vi "TWO AXIS.vi"() -> ()   [LabVIEW 2014]
uses:
  Control 1.ctl
  <vilib>/Instr/_visa.llb/VISA Flush IO Buffer Mask.ctl
  <vilib>/Instr/_visa.llb/VISA Configure Serial Port (Instr).vi
panel:
  in  "?":bool
  in  "X Positions (0<X<95)":dbl[](array[numeric])
  in  "Y Positions (0<Y<88)":dbl[](array[numeric])
  # "End Command:\n10000"
  # "There can be no values after 10000, causes the motor to rotate infinitely. To delete a cell, \nright click on the cell, then select, Data Operations -> Delete Element. \n10000 MUST BE THE LAST COMMAND."
  # "All Values are in cm."
  # "System operates by moving to a given Y-Value,\nthen iterates through all X values. After all Y-Values\nare complete the program waits for user confirmation\nthen returns to (0,0)."
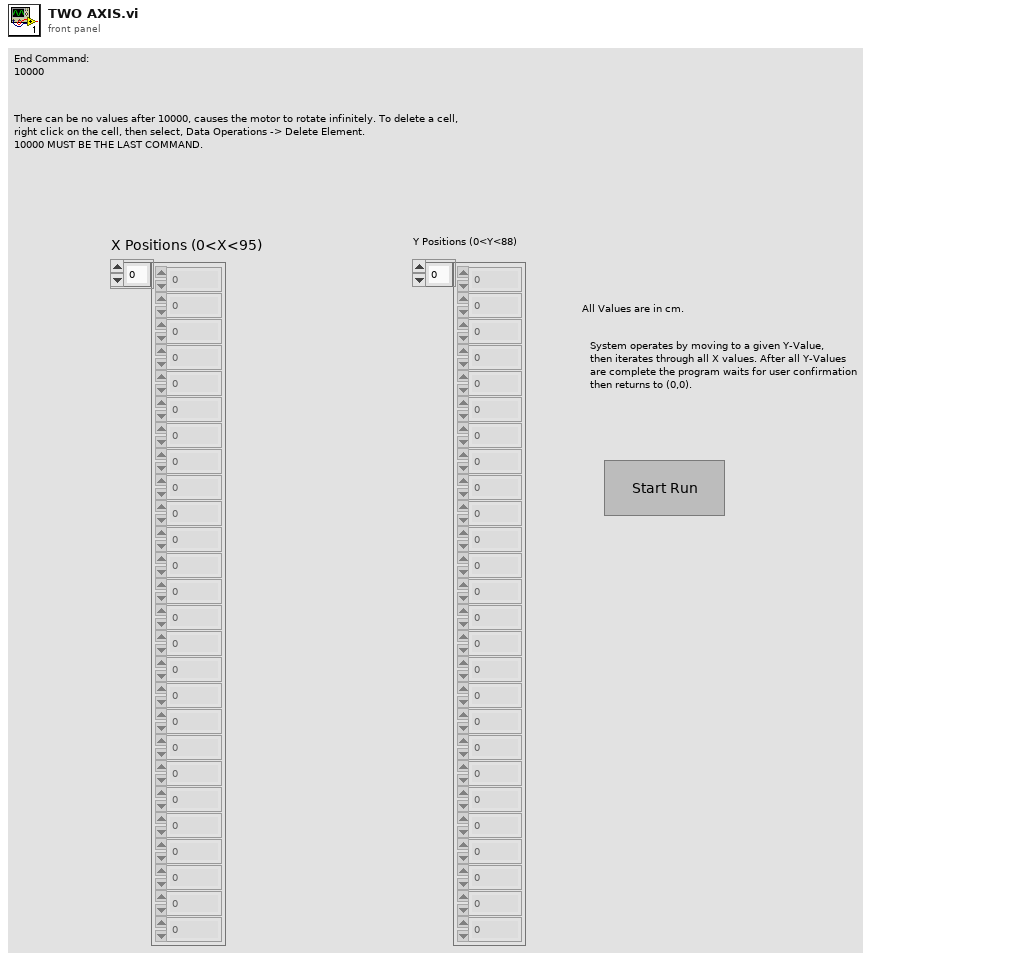
[diagram p1: front panel]
types:
  T1 = typedef "Control 1.ctl" = enum16{"Start", "Init", "Await Arduino Response", "Calculate Move", "Execute Move", "Home"}
  T2 = typedef "VISA Flush IO Buffer Mask.ctl" = u16
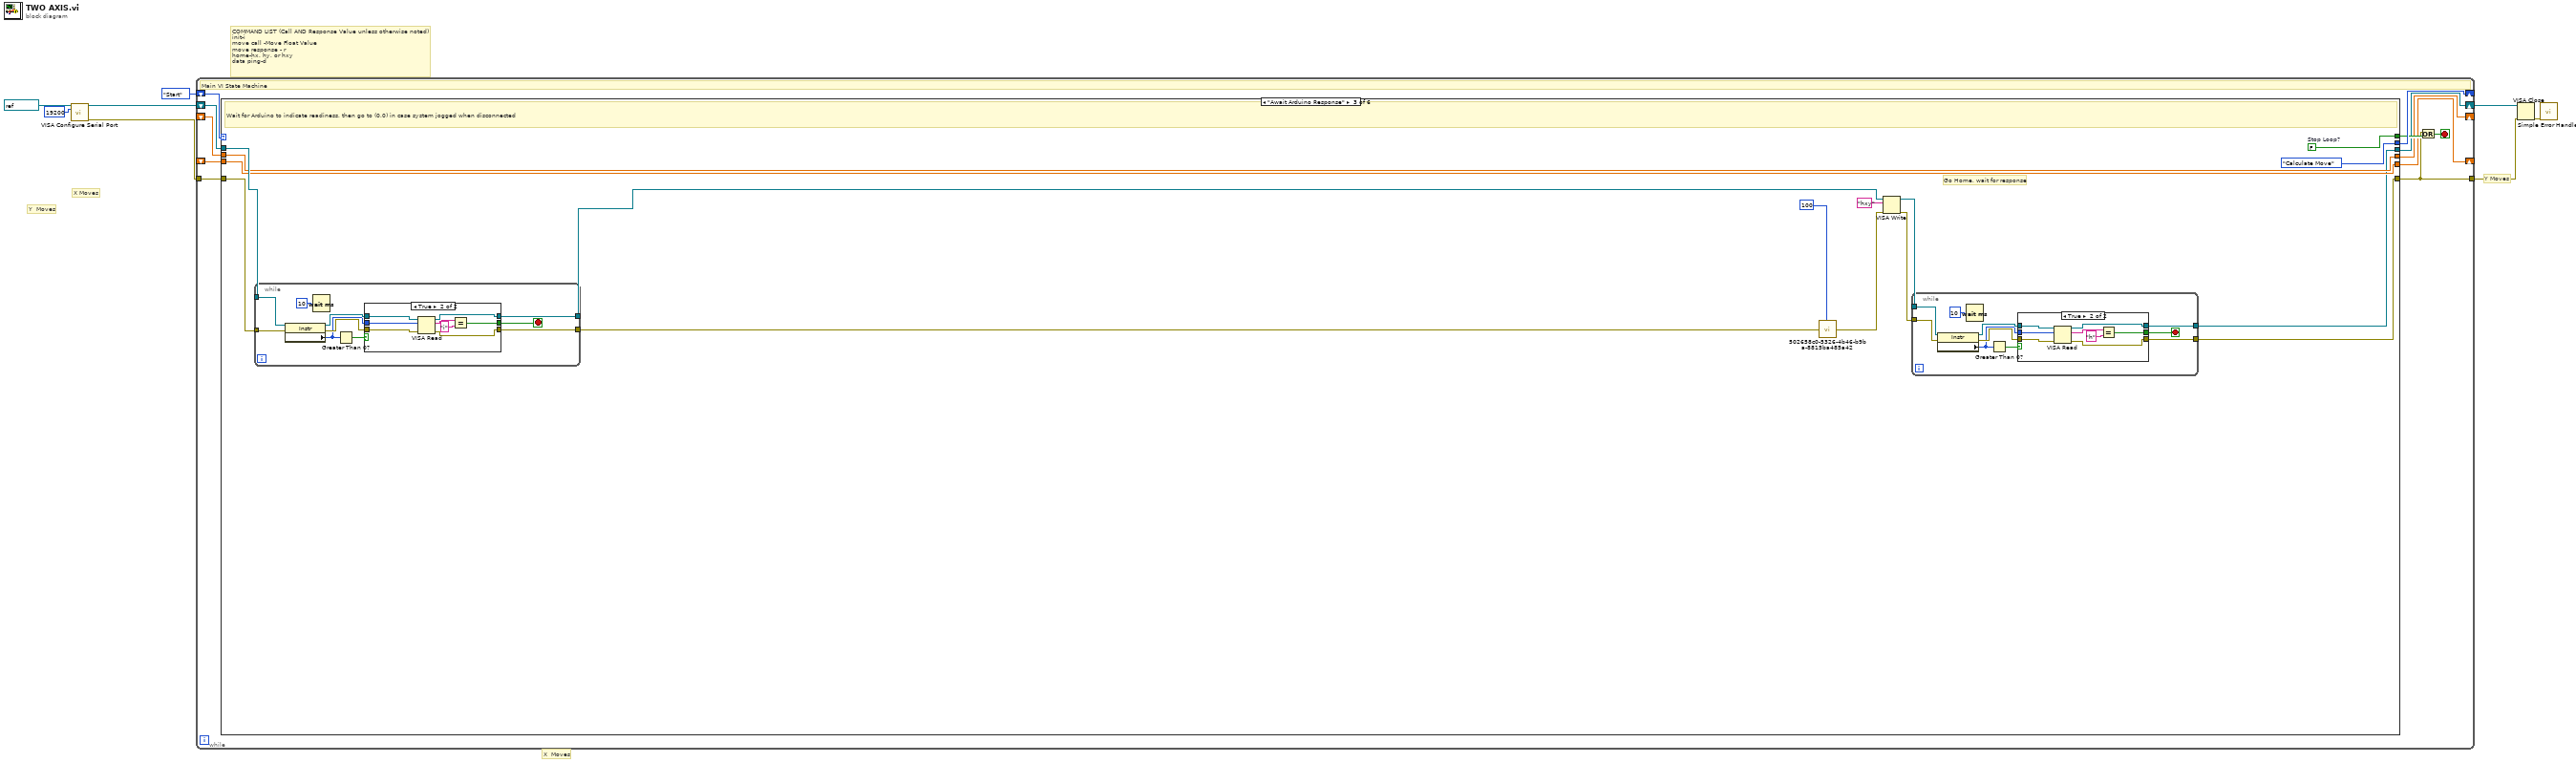
[diagram p0: block diagram]
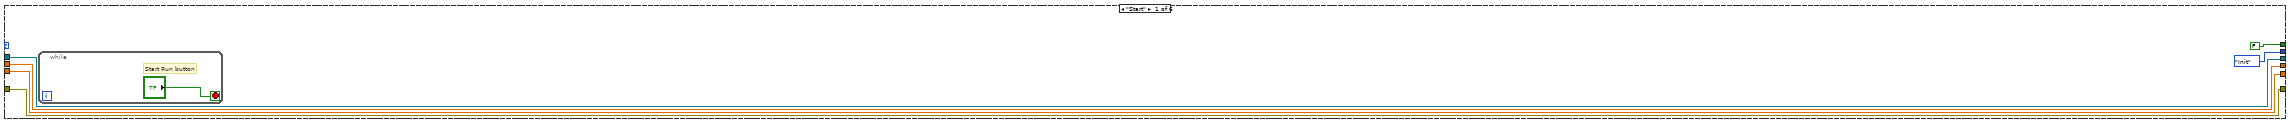
[diagram p2: hidden frame]
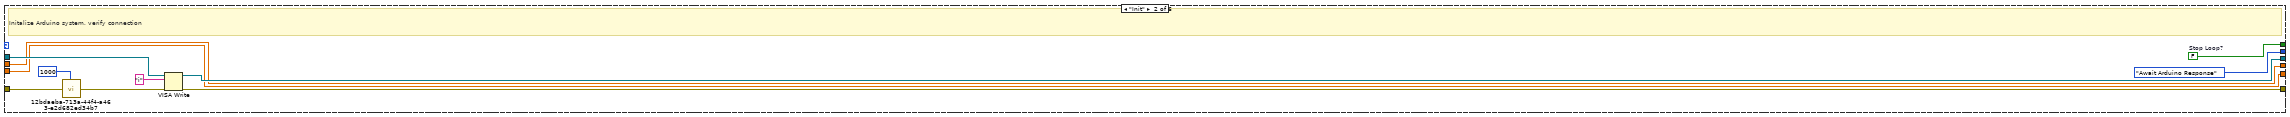
[diagram p3: hidden frame]
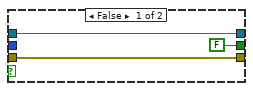
[diagram p4: hidden frame]
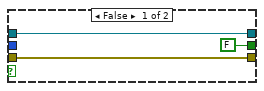
[diagram p5: hidden frame]
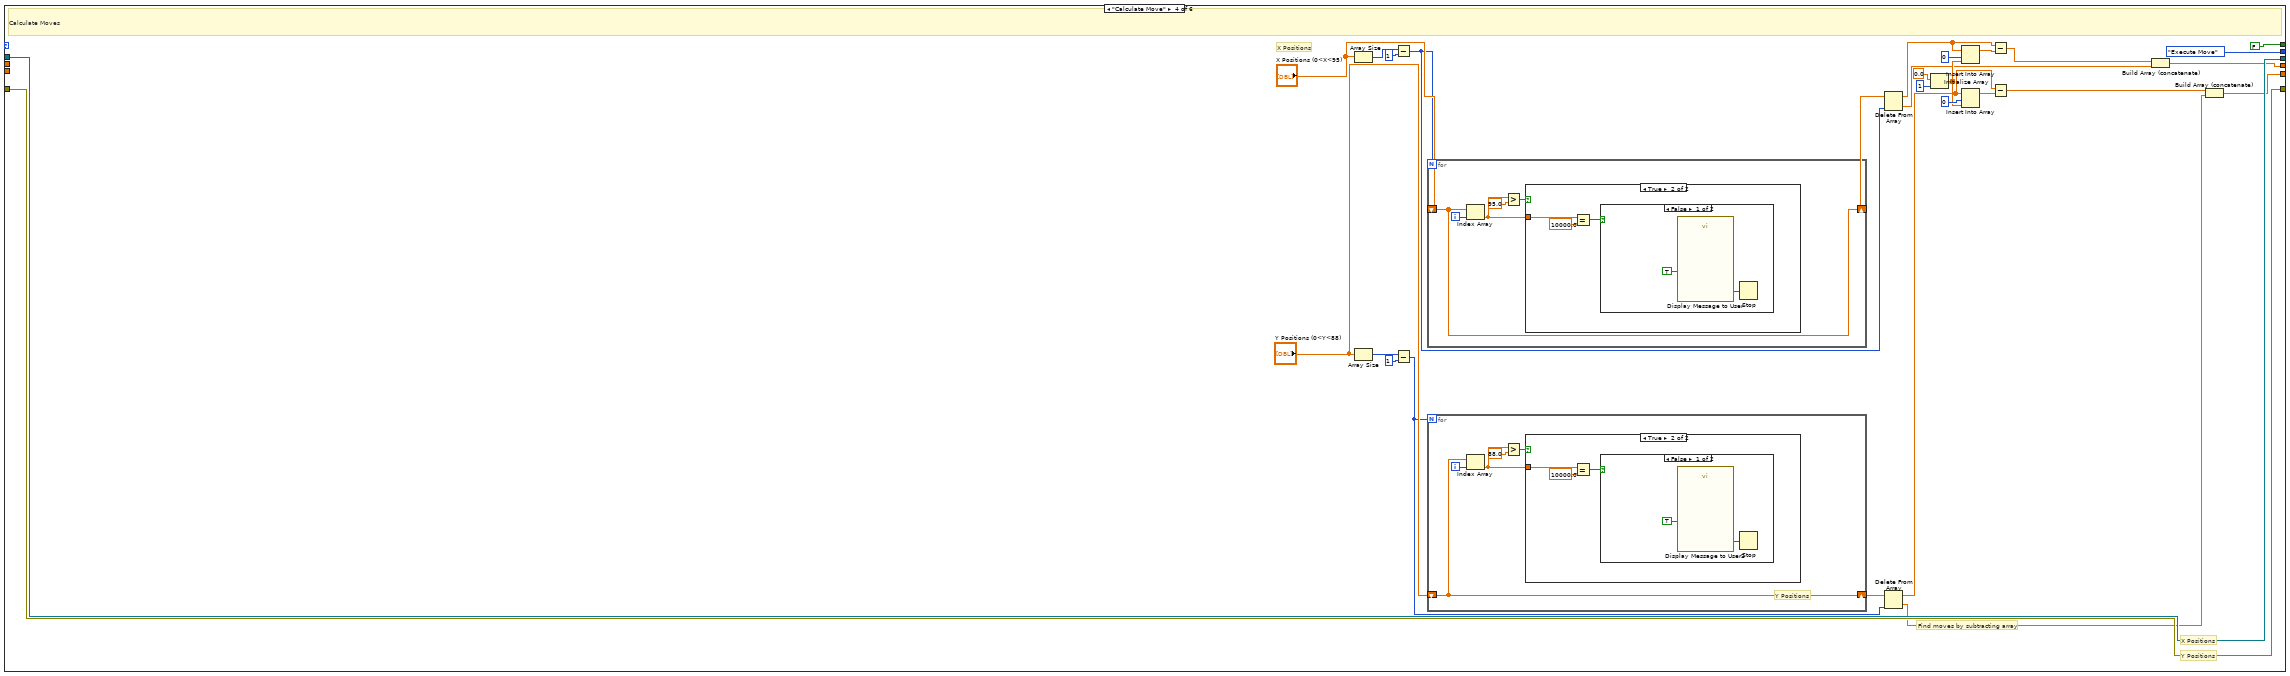
[diagram p6: hidden frame]
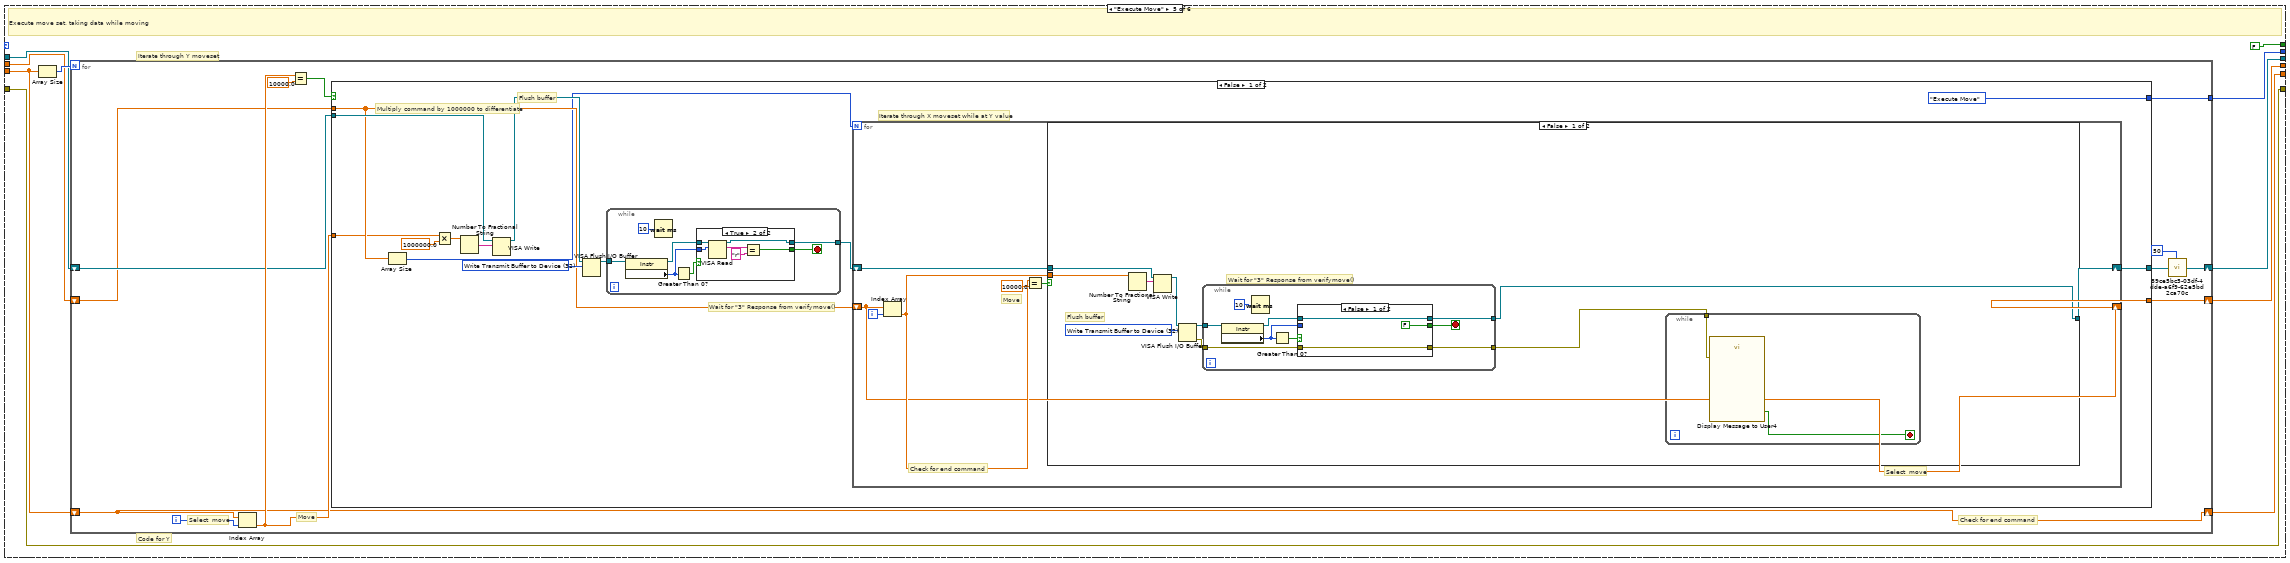
[diagram p11: hidden frame]
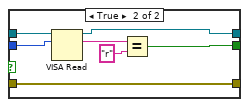
[diagram p12: hidden frame]
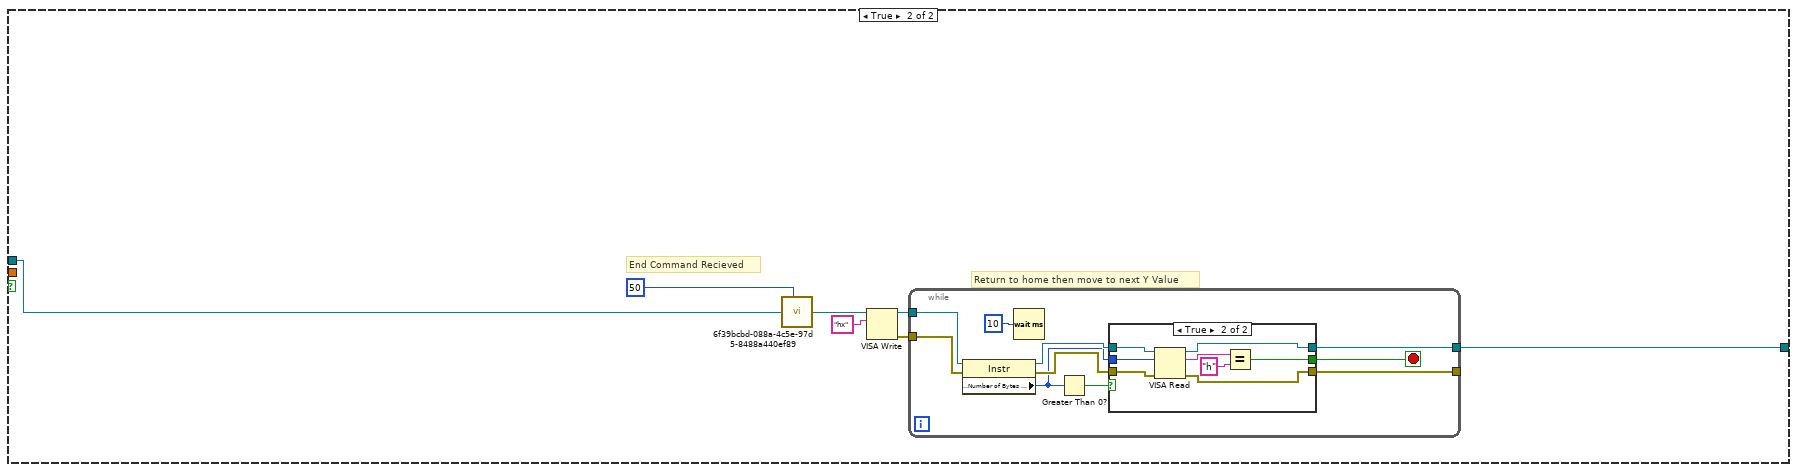
[diagram p13: hidden frame]
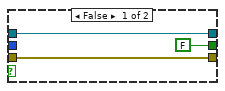
[diagram p14: hidden frame]
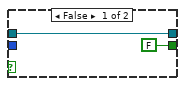
[diagram p15: hidden frame]
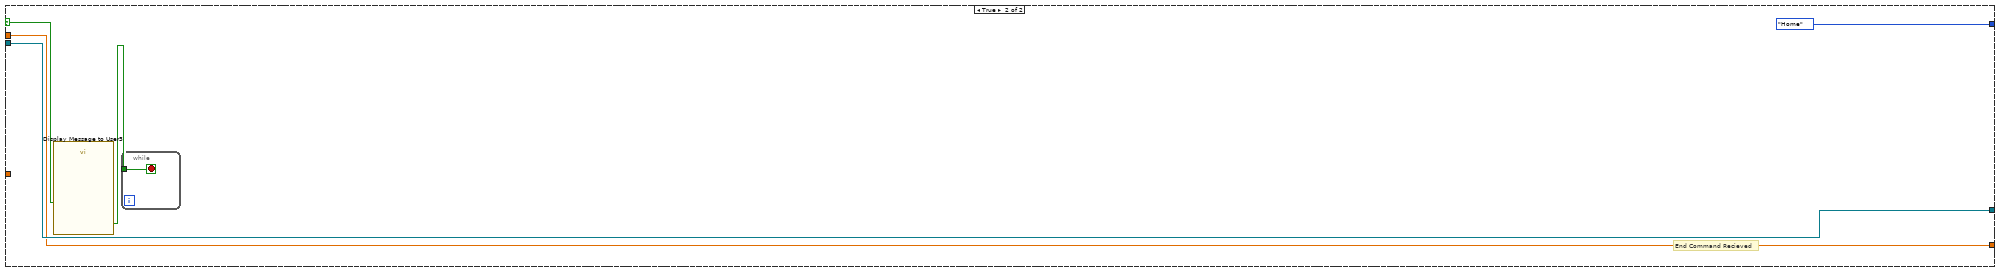
[diagram p16: hidden frame]
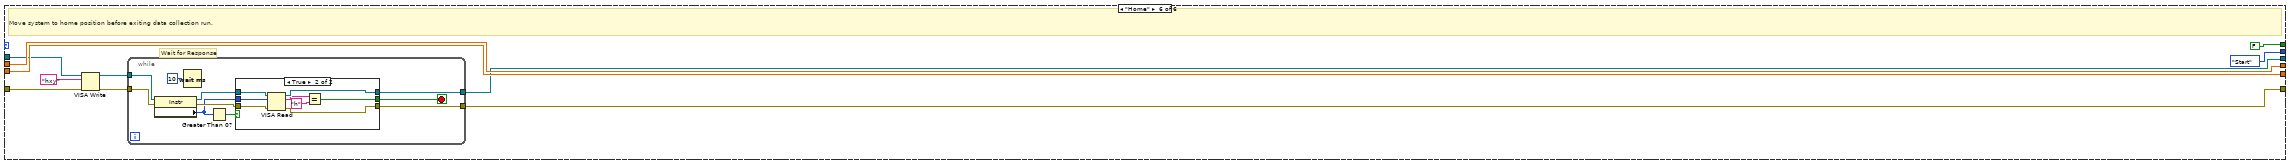
[diagram p17: hidden frame]
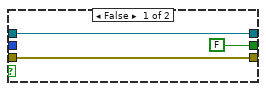
[diagram p18: hidden frame]
diagram:
  # "X  Moves"
  # "COMMAND LIST (Call AND Response Value unless otherwise noted)\ninit-i\nmove call -Move Float Value\nmove response - r\nhome-hx, hy, or hxy\ndata ping-d"
  # "Y Moves"
  # "X Moves"
  # "Y  Moves"
  n1 = call-poly "VISA Configure Serial Port"("VISA resource name"=refnum<visa-resource-name> "COM9", "baud rate (9600)"=u32 19200) -> ("VISA resource name out"=w6:refnum<visa-resource-name>, "error out"=w2:errorcluster)  [unwired: 12 in]
  n2 = while {
    shift-right: [w19] -> _
    shift-left: Control_1."Start" -> [w20]
    shift-right: [w16] -> w5
    shift-left: w6 -> [w17]
    shift-right: [w15] -> _
    shift-left: _ -> [w13]
    shift-right: [w14] -> _
    shift-left: _ -> [w12]
    tunnel: w2 -> [w11]
    tunnel: [w10] -> w1
    stop <- w9 stop-if-true
    # "Main VI State Machine"
    n3 = case shown="\"Await Arduino Response\"" w20 {
      tunnel: [Control_1."Init" Control_1."Await Arduino Response" Control_1."Calculate Move" Control_1."Execute Move" w148 Control_1."Start"] -> w19
      tunnel: [FALSE ("Stop Loop?") w38 w53 FALSE FALSE FALSE ("Stop Loop?")] -> w18
      tunnel: w17 -> [w23 w32 w52 w122 w145 w273]
      tunnel: w11 -> [w24 w34 w51 w121 w149 w272]
      tunnel: [w23 w35 w40 w122 w150 w268] -> w16
      tunnel: [w24 w36 w39 w121 w149 w267] -> w10
      tunnel: [w26 w29 w49 w104 w146 w275] -> w15
      tunnel: [w25 w28 w48 w103 w151 w274] -> w14
      tunnel: w13 -> [w26 w29 w49 _ w147 w275]
      tunnel: w12 -> [w25 w28 w48 _ w152 w274]
      frame "Start" {
        n4 = while {
          stop <- "?" stop-if-true
          # "Start Run button"
        }
      }
      frame "Init" {
        w38 = FALSE  # Stop Loop?
        # "Initalize Arduino system, verify connection"
        n5 = call "12bdaeba-713a-44f4-a463-e2d682ed34b7.vi"("value in"=w34, "milliseconds to wait"=u32 1000) -> ("value out"=w33:errorcluster)  [unwired: 1 out]
        n6 = VISA Write(VISA resource name=w32, write buffer="i", error in (no error)=w33) -> (VISA resource name out=w35:refnum<visa-resource-name>, error out=w36:errorcluster)  [unwired: 1 out]
      }
      frame "Await Arduino Response" {
        w53 = FALSE  # Stop Loop?
        # "Go Home, wait for response"
        # "Wait for Arduino to indicate readiness, then go to (0,0) in case system jogged when disconnected"
        n7 = while {
          tunnel: w52 -> [w84]
          tunnel: w51 -> [w83]
          tunnel: [w77] -> w42
          tunnel: [w76] -> w47
          stop <- w78 stop-if-true
          n8 = property class="Instr"(reference=w84, error in=w83) -> (reference out=w81:refnum<visa-resource-name>, error out=w80:errorcluster, "Serial Settings:Number of Bytes at Serial Port"=w79:u32)
          n9 = Wait (ms)(milliseconds to wait=u32 10) -> ()  [unwired: 1 out]
          n10 = Greater Than 0?(x=w79) -> (x > 0?=w82:bool)
          n11 = case shown="True" w82 {
            tunnel: w81 -> [w87 w95]
            tunnel: w80 -> [w86 w94]
            tunnel: w79 -> [_ w93]
            tunnel: [FALSE w89] -> w78
            tunnel: [w87 w91] -> w77
            tunnel: [w86 w90] -> w76
            frame False {
            }
            frame True {
              n12 = VISA Read(VISA resource name=w95, byte count=w93, error in (no error)=w94) -> (VISA resource name out=w91:refnum<visa-resource-name>, read buffer=w88:string, error out=w90:errorcluster)  [unwired: 1 out]
              n13 = Equal?(x=w88, y="i") -> (x = y?=w89:bool)
            }
          }
        }
        n14 = call "502658c0-5326-4b46-b9ba-8815ba485a42.vi"("value in"=w47, "milliseconds to wait"=u32 100) -> ("value out"=w41:errorcluster)  [unwired: 1 out]
        n15 = VISA Write(VISA resource name=w42, write buffer="hxy", error in (no error)=w41) -> (VISA resource name out=w44:refnum<visa-resource-name>, error out=w43:errorcluster)  [unwired: 1 out]
        n16 = while {
          tunnel: w44 -> [w63]
          tunnel: w43 -> [w62]
          tunnel: [w56] -> w40
          tunnel: [w55] -> w39
          stop <- w57 stop-if-true
          n17 = property class="Instr"(reference=w63, error in=w62) -> (reference out=w60:refnum<visa-resource-name>, error out=w59:errorcluster, "Serial Settings:Number of Bytes at Serial Port"=w58:u32)
          n18 = Wait (ms)(milliseconds to wait=u32 10) -> ()  [unwired: 1 out]
          n19 = Greater Than 0?(x=w58) -> (x > 0?=w61:bool)
          n20 = case shown="True" w61 {
            tunnel: w60 -> [w66 w74]
            tunnel: w59 -> [w65 w73]
            tunnel: w58 -> [_ w72]
            tunnel: [FALSE w68] -> w57
            tunnel: [w66 w70] -> w56
            tunnel: [w65 w69] -> w55
            frame False {
            }
            frame True {
              n21 = VISA Read(VISA resource name=w74, byte count=w72, error in (no error)=w73) -> (VISA resource name out=w70:refnum<visa-resource-name>, read buffer=w67:string, error out=w69:errorcluster)  [unwired: 1 out]
              n22 = Equal?(x=w67, y="h") -> (x = y?=w68:bool)
            }
          }
        }
      }
      frame "Calculate Move" {
        # "X Positions"
        # "Find moves by subtracting array"
        # "X Positions"
        # "Y Positions"
        # "Calculate Moves"
        n23 = Array Size(array="X Positions (0<X<95)") -> (size(s)=w119:i32)
        n24 = Array Size(array="Y Positions (0<Y<88)") -> (size(s)=w102:i32)
        n25 = Subtract(x=w119, y=1) -> (x-y=w96:i32)
        n26 = Subtract(x=w102, y=1) -> (x-y=w97:i32)
        n27 = for {
          N: w96 -> [_]
          shift-right: [w125] -> w98
          shift-left: "X Positions (0<X<95)" -> [w125]
          i -> [w126]
          n28 = Index Array(array=w125, index=w126) -> (element=w128:dbl)
          n29 = Greater?(x=w128, y=95.0) -> (0:w129:bool)
          n30 = case shown="True" w129 {
            tunnel: w128 -> [_ w132]
            frame False {
            }
            frame True {
              n31 = Equal?(x=w132, y=10000.0) -> (x = y?=w130:bool)
              n32 = case shown="False" w130 {
                frame False {
                  n33 = call "Display Message to User"("Enable"=TRUE) -> ("OK"=w133:bool)  [unwired: 9 in, 1 out]
                  n34 = Stop(stop? (T)=w133) -> ()
                }
                frame True {
                }
              }
            }
          }
        }
        n35 = for {
          N: w97 -> [_]
          shift-right: [w135] -> w120
          shift-left: "Y Positions (0<Y<88)" -> [w135]
          i -> [w136]
          # "Y Positions"
          n36 = Index Array(array=w135, index=w136) -> (element=w137:dbl)
          n37 = Greater?(x=w137, y=88.0) -> (0:w138:bool)
          n38 = case shown="True" w138 {
            tunnel: w137 -> [_ w142]
            frame False {
            }
            frame True {
              n39 = Equal?(x=w142, y=10000.0) -> (x = y?=w140:bool)
              n40 = case shown="False" w140 {
                frame False {
                  n41 = call "Display Message to User2"("Enable"=TRUE) -> ("OK"=w143:bool)  [unwired: 9 in, 1 out]
                  n42 = Stop(stop? (T)=w143) -> ()
                }
                frame True {
                }
              }
            }
          }
        }
        n43 = Delete From Array(array=w98, index=w96) -> (deleted portion=w105:dbl, array with subset deleted=w112:dbl[])  [unwired: 1 in]
        n44 = Delete From Array(array=w120, index=w97) -> (deleted portion=w106:dbl, array with subset deleted=w109:dbl[])  [unwired: 1 in]
        n45 = Initialize Array(0.0 ("element"), 1 ("dimension size")) -> (w113:dbl[])
        n46 = Insert Into Array(array=w112, index=0, new element=w113) -> (w111:dbl[])
        n47 = Insert Into Array(array=w109, index=0, new element=w113) -> (w110:dbl[])
        n48 = Subtract(x=w112, y=w111) -> (x-y=w108:dbl[])
        n49 = Subtract(x=w109, y=w110) -> (x-y=w107:dbl[])
        n50 = Build Array (concatenate)(w108, w105) -> (w104:dbl[])
        n51 = Build Array (concatenate)(w107, w106) -> (w103:dbl[])
      }
      frame "Execute Move" {
        # "Iterate through Y moveset"
        # "Code for Y"
        # "Execute move set, taking data while moving"
        n52 = Array Size(array=w152) -> (size(s)=w153:i32)
        n53 = for {
          N: w153 -> [_]
          shift-right: [w162] -> w151
          shift-left: w152 -> [w162]
          tunnel: [w161] -> w148
          shift-right: [w158] -> w150
          shift-left: w145 -> [w160]
          shift-right: [w155] -> w146
          shift-left: w147 -> [w156]
          i -> [w166]
          # "Select  move"
          # "Check for end command"
          # "Move"
          n54 = Index Array(array=w162, index=w166) -> (element=w163:dbl)
          n55 = Equal?(x=w163, y=10000.0) -> (x = y?=w164:bool)
          n56 = case shown="False" w164 {
            selector: w164 -> [_ w264]
            tunnel: w163 -> [w169 _]
            tunnel: [Control_1."Execute Move" Control_1."Home"] -> w161
            tunnel: w160 -> [w179 w262]
            tunnel: [w172 w262] -> w159
            tunnel: w156 -> [w171 w261]
            tunnel: [w173 w261] -> w155
            frame False {
              w175 = T2 32 items=["Flush Receive Buffer"=16, "Write Transmit Buffer to Device"=32, "Flush Receive Buffer (No I/O)"=64, "Flush Transmit Buffer"=128] ("Mask")
              # "Flush buffer"
              # "Iterate through X moveset while at Y value"
              # "Multiply command by 1000000 to differentiate"
              # "Wait for \"3\" Response from verifymove()"
              n57 = Array Size(array=w171) -> (size(s)=w170:i32)
              n58 = Multiply(x=w169, y=1000000.0) -> (x*y=w168:dbl)
              n59 = Number To Fractional String(number=w168) -> (F-format string=w178:string)  [unwired: 3 in]
              n60 = VISA Write(VISA resource name=w179, write buffer=w178) -> (VISA resource name out=w177:refnum<visa-resource-name>)  [unwired: 1 in, 2 out]
              n61 = VISA Flush I/O Buffer(VISA resource name=w177, mask (16)=w175) -> (VISA resource name out=w176:refnum<visa-resource-name>)  [unwired: 1 in, 1 out]
              n62 = while {
                tunnel: w176 -> [w252]
                tunnel: [w247] -> w174
                stop <- w248 stop-if-true
                n63 = property class="Instr"(reference=w252) -> (reference out=w250:refnum<visa-resource-name>, "Serial Settings:Number of Bytes at Serial Port"=w249:u32)  [unwired: 1 in, 1 out]
                n64 = Wait (ms)(milliseconds to wait=u32 10) -> ()  [unwired: 1 out]
                n65 = Greater Than 0?(x=w249) -> (x > 0?=w251:bool)
                n66 = case shown="True" w251 {
                  tunnel: w250 -> [w254 w260]
                  tunnel: w249 -> [_ w259]
                  tunnel: [FALSE w257] -> w248
                  tunnel: [w254 w258] -> w247
                  frame False {
                  }
                  frame True {
                    n67 = VISA Read(VISA resource name=w260, byte count=w259) -> (VISA resource name out=w258:refnum<visa-resource-name>, read buffer=w256:string)  [unwired: 1 in, 2 out]
                    n68 = Equal?(x=w256, y="r") -> (x = y?=w257:bool)
                  }
                }
              }
              n69 = for {
                N: w170 -> [_]
                shift-right: [w182] -> w173
                shift-left: w171 -> [w182]
                shift-right: [w181] -> w172
                shift-left: w174 -> [w183]
                i -> [w187]
                # "Check for end command"
                # "Move"
                # "Select  move"
                n70 = Index Array(array=w182, index=w187) -> (element=w184:dbl)
                n71 = Equal?(x=w184, y=10000.0) -> (x = y?=w185:bool)
                n72 = case shown="False" w185 {
                  tunnel: w184 -> [w195 _]
                  tunnel: w183 -> [w196 w220]
                  tunnel: [w189 w221] -> w181
                  frame False {
                    w191 = T2 32 items=["Flush Receive Buffer"=16, "Write Transmit Buffer to Device"=32, "Flush Receive Buffer (No I/O)"=64, "Flush Transmit Buffer"=128] ("Mask")
                    # "Flush buffer"
                    # "Wait for \"3\" Response from verifymove()"
                    n73 = Number To Fractional String(number=w195) -> (F-format string=w194:string)  [unwired: 3 in]
                    n74 = VISA Write(VISA resource name=w196, write buffer=w194) -> (VISA resource name out=w193:refnum<visa-resource-name>)  [unwired: 1 in, 2 out]
                    n75 = VISA Flush I/O Buffer(VISA resource name=w193, mask (16)=w191) -> (VISA resource name out=w192:refnum<visa-resource-name>, error out=w190:errorcluster)  [unwired: 1 in]
                    n76 = while {
                      tunnel: w192 -> [w207]
                      tunnel: [w202] -> w189
                      tunnel: w190 -> [w200]
                      tunnel: [w199] -> w188
                      stop <- w203 stop-if-true
                      n77 = property class="Instr"(reference=w207) -> (reference out=w205:refnum<visa-resource-name>, "Serial Settings:Number of Bytes at Serial Port"=w204:u32)  [unwired: 1 in, 1 out]
                      n78 = Wait (ms)(milliseconds to wait=u32 10) -> ()  [unwired: 1 out]
                      n79 = Greater Than 0?(x=w204) -> (x > 0?=w206:bool)
                      n80 = case shown="False" w206 {
                        tunnel: w205 -> [w210 w217]
                        tunnel: w204 -> [_ w216]
                        tunnel: [FALSE w214] -> w203
                        tunnel: [w210 w215] -> w202
                        tunnel: w200 -> [w208 w211]
                        tunnel: [w208 w211] -> w199
                        frame False {
                        }
                        frame True {
                          n81 = VISA Read(VISA resource name=w217, byte count=w216) -> (VISA resource name out=w215:refnum<visa-resource-name>, read buffer=w213:string)  [unwired: 1 in, 2 out]
                          n82 = Equal?(x=w213, y="r") -> (x = y?=w214:bool)
                        }
                      }
                    }
                    n83 = while {
                      tunnel: w188 -> [w198]
                      stop <- w197 stop-if-true
                      n84 = call "Display Message to User4"("error in (no error)"=w198) -> ("Continue"=w197:bool)  [unwired: 9 in, 1 out]
                    }
                  }
                  frame True {
                    # "Return to home then move to next Y Value"
                    # "End Command Recieved"
                    n85 = call "6f39bcbd-088a-4c5e-97d5-8488a440ef89.vi"("value in"=w220, "milliseconds to wait"=u32 50) -> ("value out"=w219:refnum<visa-resource-name>)  [unwired: 1 out]
                    n86 = VISA Write(VISA resource name=w219, write buffer="hx") -> (VISA resource name out=w223:refnum<visa-resource-name>, error out=w222:errorcluster)  [unwired: 1 in, 1 out]
                    n87 = while {
                      tunnel: w223 -> [w234]
                      tunnel: w222 -> [w233]
                      tunnel: [w227] -> w221
                      tunnel: [w226] -> _
                      stop <- w228 stop-if-true
                      n88 = property class="Instr"(reference=w234, error in=w233) -> (reference out=w231:refnum<visa-resource-name>, error out=w230:errorcluster, "Serial Settings:Number of Bytes at Serial Port"=w229:u32)
                      n89 = Wait (ms)(milliseconds to wait=u32 10) -> ()  [unwired: 1 out]
                      n90 = Greater Than 0?(x=w229) -> (x > 0?=w232:bool)
                      n91 = case shown="True" w232 {
                        tunnel: w231 -> [w237 w245]
                        tunnel: w230 -> [w236 w244]
                        tunnel: w229 -> [_ w243]
                        tunnel: [FALSE w239] -> w228
                        tunnel: [w237 w241] -> w227
                        tunnel: [w236 w240] -> w226
                        frame False {
                        }
                        frame True {
                          n92 = VISA Read(VISA resource name=w245, byte count=w243, error in (no error)=w244) -> (VISA resource name out=w241:refnum<visa-resource-name>, read buffer=w238:string, error out=w240:errorcluster)  [unwired: 1 out]
                          n93 = Equal?(x=w238, y="h") -> (x = y?=w239:bool)
                        }
                      }
                    }
                  }
                }
              }
            }
            frame True {
              # "End Command Recieved"
              n94 = call "Display Message to User3"("Enable"=w264) -> ("Return to Home"=w265:bool)  [unwired: 9 in, 1 out]
              n95 = while {
                tunnel: w265 -> [w266]
                stop <- w266 stop-if-true
              }
            }
          }
          n96 = call "89ce5bc5-03df-4dde-a6f9-62e5bd2ca70c.vi"("value in"=w159, "milliseconds to wait"=u32 50) -> ("value out"=w158:refnum<visa-resource-name>)  [unwired: 1 out]
        }
      }
      frame "Home" {
        # "Wait for Response"
        # "Move system to home position before exiting data collection run."
        n97 = VISA Write(VISA resource name=w273, write buffer="hxy", error in (no error)=w272) -> (VISA resource name out=w270:refnum<visa-resource-name>, error out=w269:errorcluster)  [unwired: 1 out]
        n98 = while {
          tunnel: w270 -> [w287]
          tunnel: w269 -> [w286]
          tunnel: [w280] -> w268
          tunnel: [w279] -> w267
          stop <- w281 stop-if-true
          n99 = property class="Instr"(reference=w287, error in=w286) -> (reference out=w284:refnum<visa-resource-name>, error out=w283:errorcluster, "Serial Settings:Number of Bytes at Serial Port"=w282:u32)
          n100 = Wait (ms)(milliseconds to wait=u32 10) -> ()  [unwired: 1 out]
          n101 = Greater Than 0?(x=w282) -> (x > 0?=w285:bool)
          n102 = case shown="True" w285 {
            tunnel: w284 -> [w290 w298]
            tunnel: w283 -> [w289 w297]
            tunnel: w282 -> [_ w296]
            tunnel: [FALSE w292] -> w281
            tunnel: [w290 w294] -> w280
            tunnel: [w289 w293] -> w279
            frame False {
            }
            frame True {
              n103 = VISA Read(VISA resource name=w298, byte count=w296, error in (no error)=w297) -> (VISA resource name out=w294:refnum<visa-resource-name>, read buffer=w291:string, error out=w293:errorcluster)  [unwired: 1 out]
              n104 = Equal?(x=w291, y="h") -> (x = y?=w292:bool)
            }
          }
        }
      }
    }
    n105 = Or(x=w10, y=w18) -> (x .or. y?=w9:bool)
  }
  n106 = VISA Close(VISA resource name=w5, error in (no error)=w1) -> (error out=w7:errorcluster)
  n107 = call <vilib>:"Simple Error Handler.vi"("error in (no error)"=w7) -> ()  [unwired: 4 in, 5 out]
